vi "Create DocumentTag.vi"(8 "error in (no error)":errorcluster, 9 "Generate Help Tag W":bool, 10 "Name":string, 11 "Help:Document Tag W":refnum<vi>) -> (0 "error out":errorcluster)   [LabVIEW 2020]
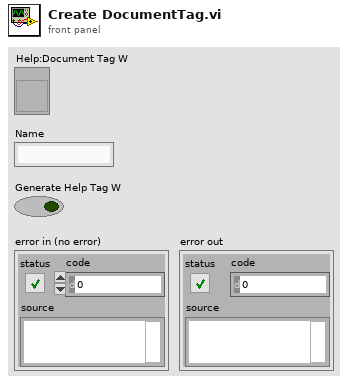
[diagram p1: front panel]
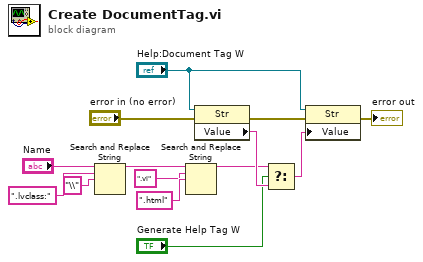
[diagram p0: block diagram]
diagram:
  n1 = Search and Replace String(input string="Name", search string=".lvclass:", replace string="\\" ("replace string (\"\")")) -> (result string=w6:string)  [unwired: 5 in, 3 out]
  n2 = Search and Replace String(input string=w6, search string=".vi", replace string=".html" ("search string")) -> (result string=w9:string)  [unwired: 5 in, 3 out]
  n3 = property on="Property Node" class="Str"(reference="Help:Document Tag W", error in="error in (no error)") -> (error out=w13:errorcluster, "Value"=w14:string)  [unwired: 1 out]
  n4 = Select(t=w9, s="Generate Help Tag W", f=w14) -> (s? t:f=w5:string)
  n5 = property on="Property Node" class="Str"(reference="Help:Document Tag W", error in=w13, "Value"=w5) -> (error out=→"error out":errorcluster)  [unwired: 1 out]
